vi "Fault_Table_Read.vi"(7 "ERD Data Out":cluster{"ERD Number":u16, "Data":string}[](array[cluster]) {"ERD Number" format="%.0x"}) -> (1 "Fault Set?":bool, 2 "Table Buffer Status":T3, 3 "Fault Table String Out":string[][](array[string]), 4 "Fault Table Array Out":T1)   [LabVIEW 2016]
uses:
  Type Definitions/2015 Program/Fault_Buffer_Status.ctl
  Type Definitions/2015 Program/Fault Table Array.ctl
  Washer Soft Load Box/type defs/Fault_Table_Info.ctl
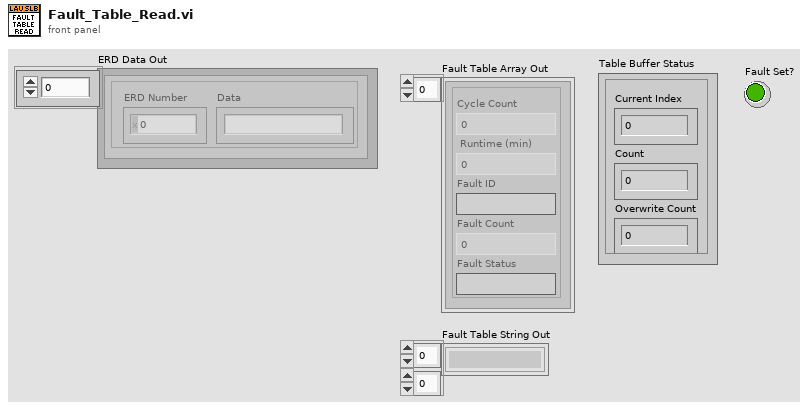
[diagram p1: front panel]
types:
  T1 = typedef "Fault Table Array.ctl" = T2[]
  T2 = typedef "Fault_Table_Info.ctl" = cluster{"Cycle Count":u32, " Runtime (min) ":u32, "Fault Status":string, "Fault ID":string, "Fault Count":u16}
  T3 = typedef "Fault_Buffer_Status.ctl" = cluster{"Current Index":u16, "Count":u16, "Overwrite Count":u16}
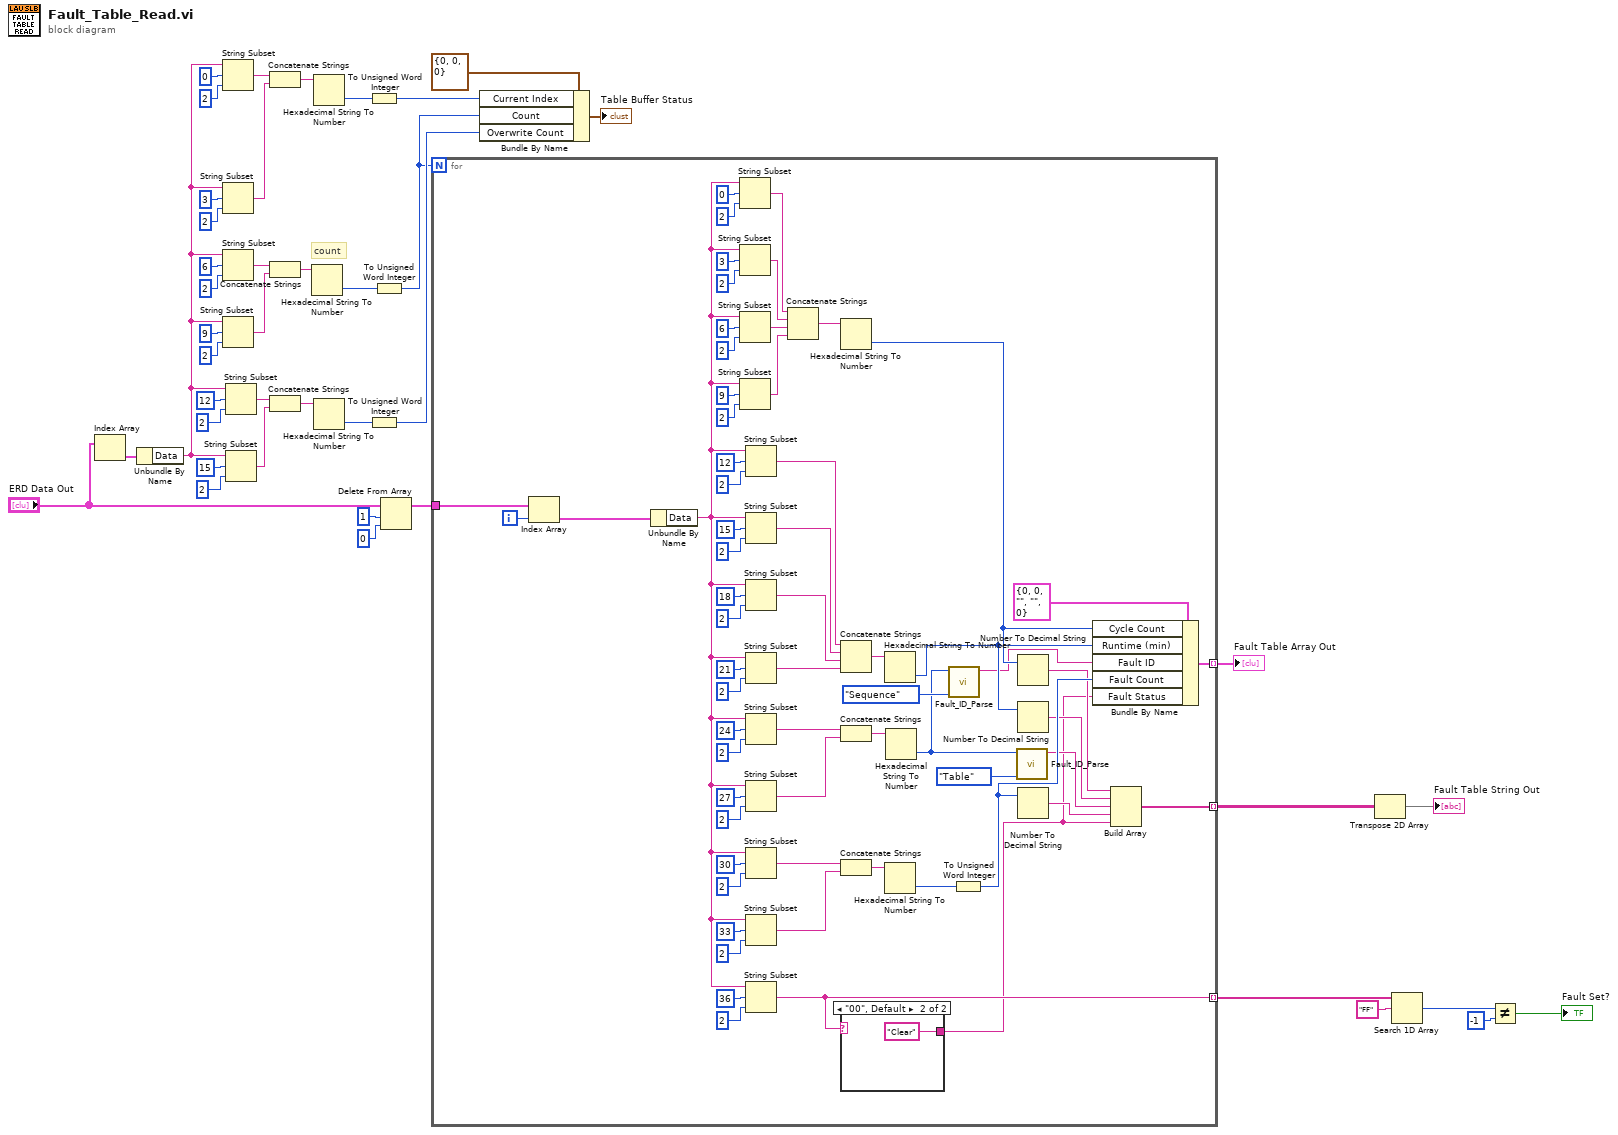
[diagram p0: block diagram]
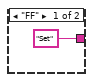
[diagram p2: hidden frame]
diagram:
  # "count"
  n1 = Index Array(array="ERD Data Out") -> (element=w36:cluster{"ERD Number":u16, "Data":string})  [unwired: 1 in]
  n2 = Unbundle By Name(w36) -> ("Data"=w15:string)
  n3 = String Subset(string=w15, offset (0)=0, length (rest)=2 ("length (rest)")) -> (substring=w24:string)
  n4 = String Subset(string=w15, offset (0)=3, length (rest)=2 ("length (rest)")) -> (substring=w25:string)
  n5 = String Subset(string=w15, offset (0)=6, length (rest)=2 ("length (rest)")) -> (substring=w40:string)
  n6 = String Subset(string=w15, offset (0)=9, length (rest)=2 ("length (rest)")) -> (substring=w39:string)
  n7 = String Subset(string=w15, offset (0)=12, length (rest)=2 ("length (rest)")) -> (substring=w26:string)
  n8 = String Subset(string=w15, offset (0)=15, length (rest)=2 ("length (rest)")) -> (substring=w27:string)
  n9 = Concatenate Strings(w24, w25) -> (w28:string)
  n10 = Concatenate Strings(w40, w39) -> (w38:string)
  n11 = Concatenate Strings(w26, w27) -> (w29:string)
  n12 = Hexadecimal String To Number(string=w38) -> (number=w37:u32)  [unwired: 2 in, 1 out]
  n13 = Hexadecimal String To Number(string=w28) -> (number=w31:u32)  [unwired: 2 in, 1 out]
  n14 = Hexadecimal String To Number(string=w29) -> (number=w32:u32)  [unwired: 2 in, 1 out]
  n15 = To Unsigned Word Integer(number=w31) -> (unsigned 16bit integer=w33:u16)
  n16 = To Unsigned Word Integer(number=w32) -> (unsigned 16bit integer=w34:u16)
  n17 = To Unsigned Word Integer(number=w37) -> (unsigned 16bit integer=w8:u16)
  n18 = Delete From Array(array="ERD Data Out", length=1, index=0) -> (array with subset deleted=w5:cluster{"ERD Number":u16, "Data":string}[])  [unwired: 1 out]
  n19 = for {
    N: w8 -> [_]
    tunnel: [w61] -> w1 mode=indexing
    tunnel: [w59] -> w13 mode=indexing
    tunnel: w5 -> [w57]
    tunnel: [w48] -> w3 mode=indexing
    i -> [w58]
    n20 = Index Array(array=w57, index=w58) -> (element=w60:cluster{"ERD Number":u16, "Data":string})
    n21 = Unbundle By Name(w60) -> ("Data"=w66:string)
    n22 = String Subset(string=w66, offset (0)=0, length (rest)=2 ("length (rest)")) -> (substring=w101:string)
    n23 = String Subset(string=w66, offset (0)=3, length (rest)=2 ("length (rest)")) -> (substring=w100:string)
    n24 = String Subset(string=w66, offset (0)=6, length (rest)=2 ("length (rest)")) -> (substring=w99:string)
    n25 = String Subset(string=w66, offset (0)=9, length (rest)=2 ("length (rest)")) -> (substring=w98:string)
    n26 = String Subset(string=w66, offset (0)=12, length (rest)=2 ("length (rest)")) -> (substring=w92:string)
    n27 = String Subset(string=w66, offset (0)=15, length (rest)=2 ("length (rest)")) -> (substring=w93:string)
    n28 = String Subset(string=w66, offset (0)=18, length (rest)=2 ("length (rest)")) -> (substring=w94:string)
    n29 = String Subset(string=w66, offset (0)=21, length (rest)=2 ("length (rest)")) -> (substring=w95:string)
    n30 = String Subset(string=w66, offset (0)=24, length (rest)=2 ("length (rest)")) -> (substring=w85:string)
    n31 = String Subset(string=w66, offset (0)=27, length (rest)=2 ("length (rest)")) -> (substring=w84:string)
    n32 = String Subset(string=w66, offset (0)=30, length (rest)=2 ("length (rest)")) -> (substring=w64:string)
    n33 = String Subset(string=w66, offset (0)=33, length (rest)=2 ("length (rest)")) -> (substring=w63:string)
    n34 = String Subset(string=w66, offset (0)=36, length (rest)=2 ("length (rest)")) -> (substring=w59:string)
    n35 = Concatenate Strings(w101, w100, w99, w98) -> (w97:string)
    n36 = Hexadecimal String To Number(string=w97) -> (number=w56:u32)  [unwired: 2 in, 1 out]
    n37 = Concatenate Strings(w92, w93, w94, w95) -> (w96:string)
    n38 = Concatenate Strings(w85, w84) -> (w83:string)
    n39 = Concatenate Strings(w64, w63) -> (w65:string)
    n40 = case shown="\"00\", Default" w59 {
      tunnel: ["Set" "Clear"] -> w49
      frame "FF" {
      }
      frame "00", Default {
      }
    }
    n41 = Hexadecimal String To Number(string=w96) -> (number=w55:u32)  [unwired: 2 in, 1 out]
    n42 = Hexadecimal String To Number(string=w65) -> (number=w62:u32)  [unwired: 2 in, 1 out]
    n43 = Hexadecimal String To Number(string=w83) -> (number=w45:u32)  [unwired: 2 in, 1 out]
    n44 = call "Fault_ID_Parse.vi"("Enum"=enum16{"Sequence", "Table"}."Sequence", "Numeric"=w45) -> ("String"=w44:string)  [unwired: 9 in]
    n45 = To Unsigned Word Integer(number=w62) -> (unsigned 16bit integer=w54:u16)
    n46 = call "Fault_ID_Parse.vi"("Enum"=enum16{"Sequence", "Table"}."Table", "Numeric"=w45) -> ("String"=w51:string)  [unwired: 9 in]
    n47 = Number To Decimal String(number=w56) -> (decimal integer string=w53:string)  [unwired: 1 in]
    n48 = Number To Decimal String(number=w55) -> (decimal integer string=w52:string)  [unwired: 1 in]
    n49 = Number To Decimal String(number=w54) -> (decimal integer string=w50:string)  [unwired: 1 in]
    n50 = Bundle By Name(cluster=T2 {"Cycle Count"=0, " Runtime (min) "=0, "Fault Status"="", "Fault ID"="", "Fault Count"=0} ("Fault Table 0"), "Cycle Count"=w56, "Runtime (min)"=w55, "Fault ID"=w44, "Fault Count"=w54, "Fault Status"=w49) -> (w61:T2)
    n51 = Build Array(w53, w52, w51, w50, w49) -> (w48:string[])
  }
  "Fault Table Array Out" <- w1
  n52 = Bundle By Name(cluster=T3 {"Current Index"=0, "Count"=0, "Overwrite Count"=0} ("Buffer Status"), "Current Index"=w33, "Count"=w8, "Overwrite Count"=w34) -> (→"Table Buffer Status":T3)
  n53 = Transpose 2D Array(2D array=w3) -> (transposed array=→"Fault Table String Out":string[][])
  n54 = Search 1D Array(1D array=w13, element="FF") -> (index of element=w11:i32)  [unwired: 1 in]
  n55 = Not Equal?(x=w11, y=-1) -> (x != y?=→"Fault Set?":bool)
